vi "pm.vi"() -> ()   [LabVIEW 2017]
uses:
  lowest_col.vi
  index.vi
panel:
  out "String":string
  out "Numeric 2":dbl
  out "Numeric":dbl
  in  "Array":dbl[][](array[numeric])
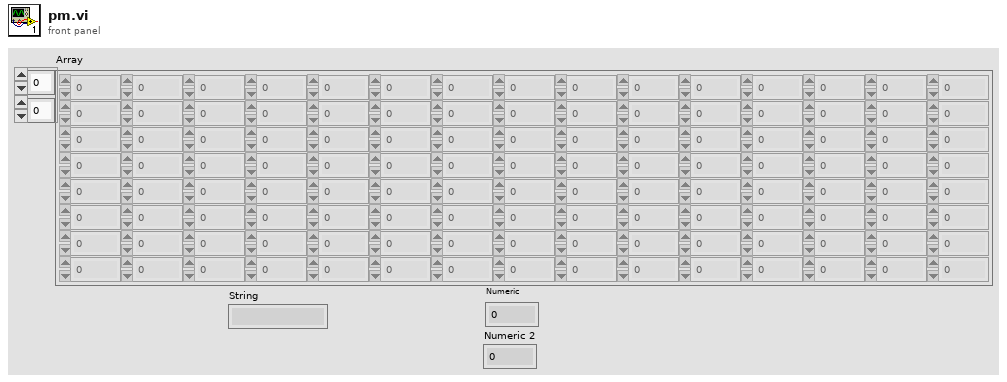
[diagram p1: front panel]
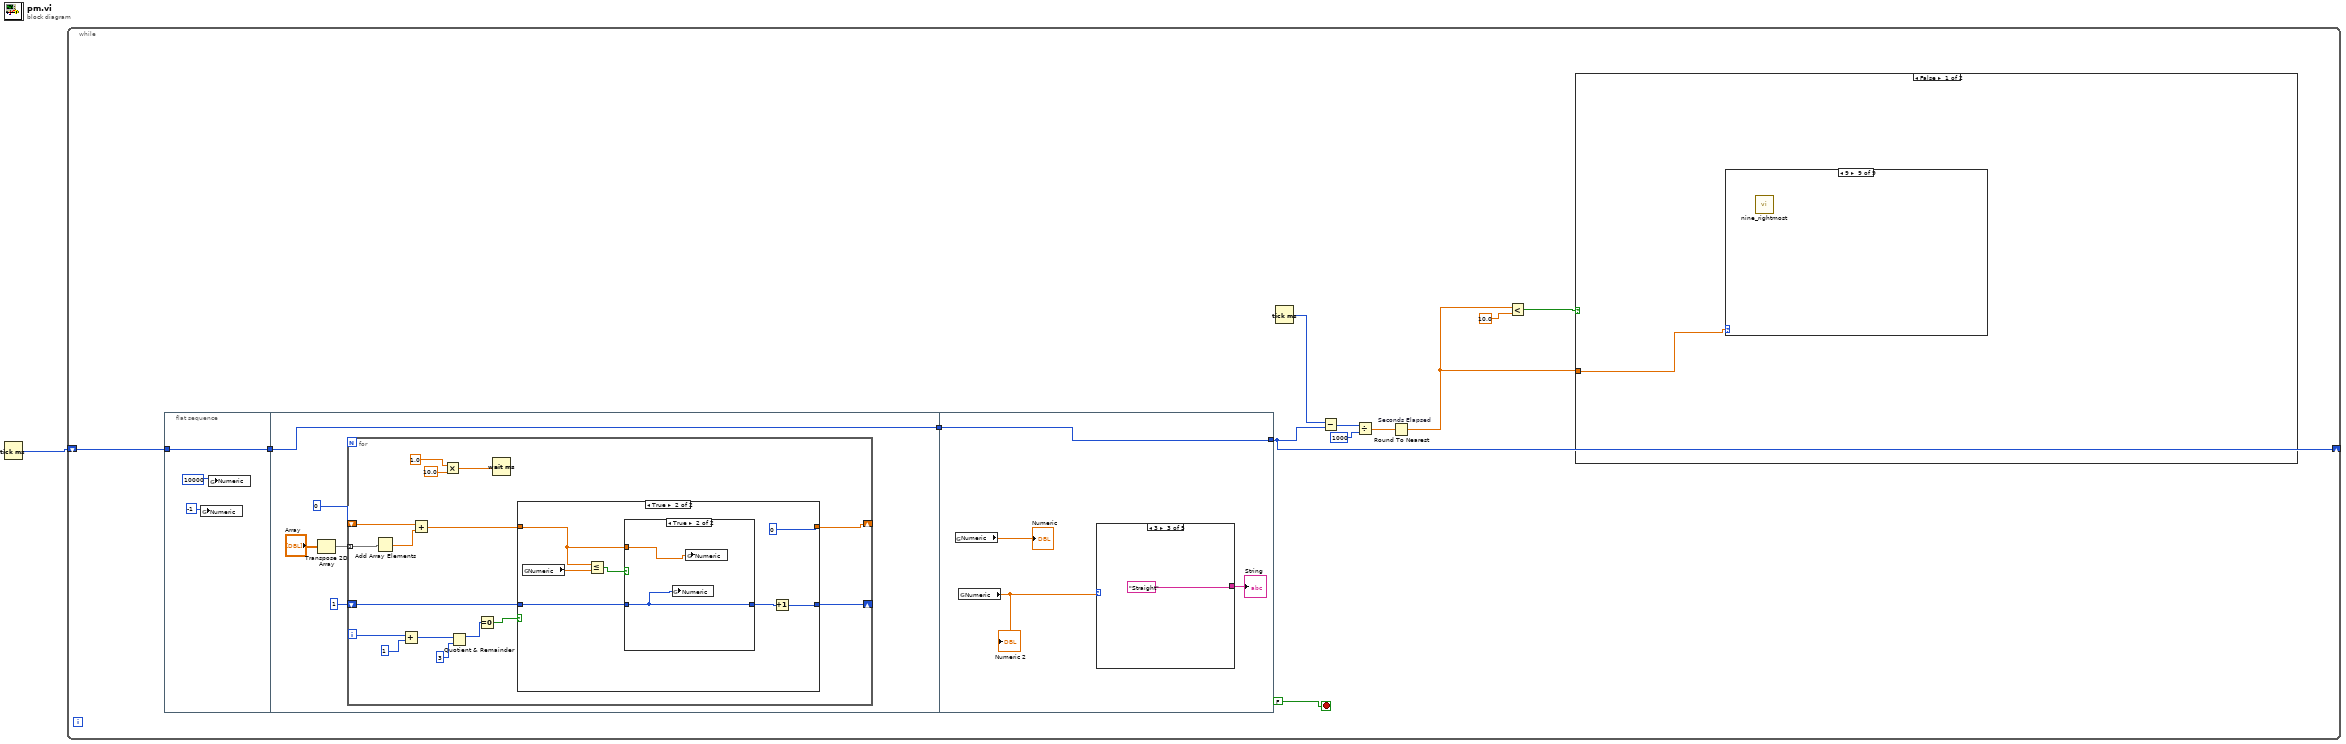
[diagram p0: block diagram]
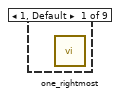
[diagram p2: hidden frame]
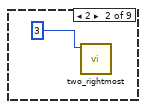
[diagram p3: hidden frame]
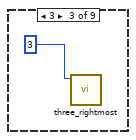
[diagram p4: hidden frame]
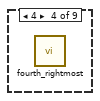
[diagram p5: hidden frame]
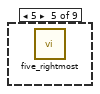
[diagram p6: hidden frame]
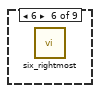
[diagram p7: hidden frame]
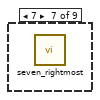
[diagram p8: hidden frame]
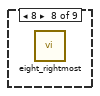
[diagram p9: hidden frame]
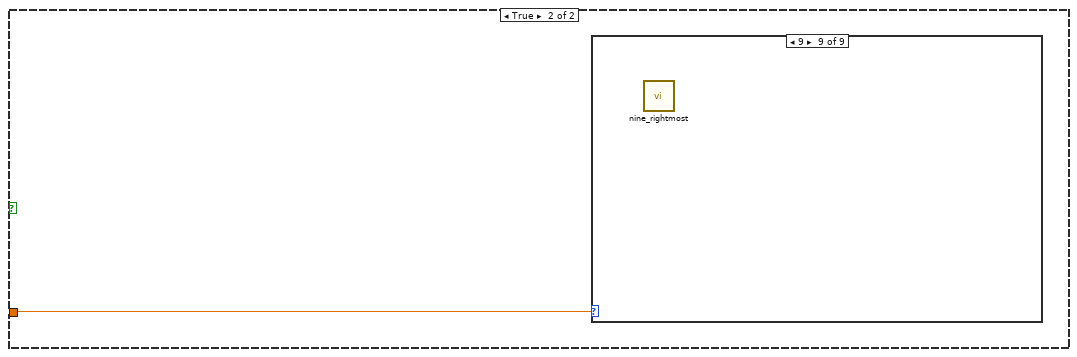
[diagram p10: hidden frame]
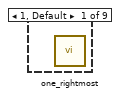
[diagram p11: hidden frame]
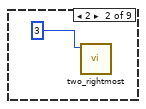
[diagram p12: hidden frame]
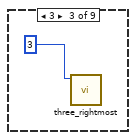
[diagram p13: hidden frame]
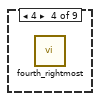
[diagram p14: hidden frame]
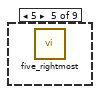
[diagram p15: hidden frame]
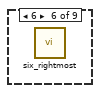
[diagram p16: hidden frame]
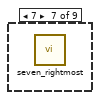
[diagram p17: hidden frame]
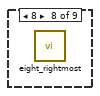
[diagram p18: hidden frame]
diagram:
  n1 = Tick Count (ms)() -> (millisecond timer value=w1:u32)
  n2 = while {
    shift-right: [w8] -> _
    shift-left: w1 -> [w10]
    stop <- FALSE stop-if-true
    n3 = flat-sequence {
      tunnel: [w20] -> w11
      tunnel: w10 -> [w20]
      tunnel: [w23] -> w12
      tunnel: w11 -> [w23]
      tunnel: [w56] -> w8
      tunnel: w12 -> [w56]
      frame #0 {
        n4 = global write "index.vi" "Numeric"(-1) -> ()
        n5 = global write "lowest_col.vi" "Numeric"(10000) -> ()
      }
      frame #1 {
        n6 = Transpose 2D Array(2D array="Array") -> (transposed array=w26:dbl[][])
        n7 = for {
          tunnel: w26 -> [w41] mode=indexing
          shift-right: [w31] -> _
          shift-left: 0 -> [w39]
          shift-right: [w28] -> _
          shift-left: 1 -> [w29]
          i -> [w38]
          n8 = Add Array Elements(numeric array=w41) -> (sum=w40:dbl)
          n9 = Add(x=w38, y=1) -> (x+y=w36:i32)
          n10 = Add(x=w39, y=w40) -> (x+y=w32:dbl)
          n11 = Multiply(x=1.0 ("number (0 to 1)"), y=10.0) -> (x*y=w42:dbl)
          n12 = Quotient & Remainder(x=w36, y=3) -> (x-y*floor(x/y)=w34:i32)  [unwired: 1 out]
          n13 = Equal To 0?(x=w34) -> (x = 0?=w33:bool)
          n14 = Wait (ms)(milliseconds to wait=w42) -> ()  [unwired: 1 out]
          n15 = case shown="True" w33 {
            tunnel: w32 -> [w45 w49]
            tunnel: [w45 0] -> w31
            tunnel: w29 -> [w44 w48]
            tunnel: [w44 w46] -> w28
            frame False {
            }
            frame True {
              n16 = global read "lowest_col.vi" "Numeric"() -> (w51:dbl)
              n17 = Less Or Equal?(x=w49, y=w51) -> (x <= y?=w50:bool)
              n18 = case shown="True" w50 {
                tunnel: w49 -> [_ w55]
                tunnel: w48 -> [w53 w54]
                tunnel: [w53 w54] -> w47
                frame False {
                }
                frame True {
                  n19 = global write "index.vi" "Numeric"(w54) -> ()
                  n20 = global write "lowest_col.vi" "Numeric"(w55) -> ()
                }
              }
              n21 = Increment(x=w47) -> (x+1=w46:i32)
            }
          }
        }
      }
      frame #2 {
        n22 = global read "lowest_col.vi" "Numeric"() -> (→"Numeric":dbl)
        n23 = global read "index.vi" "Numeric"() -> (w58:dbl)
        "Numeric 2" <- w58
        n24 = case shown="3" w58 {
          tunnel: ["Hard Left" "Soft Left" "Straight" "Soft Right" "Hard Right"] -> w57
          frame 1, Default {
          }
          frame 2 {
          }
          frame 3 {
          }
          frame 4 {
          }
          frame 5 {
          }
        }
        "String" <- w57
      }
    }
    n25 = Tick Count (ms)() -> (millisecond timer value=w9:u32)
    n26 = Subtract(x=w9, y=w8) -> (x-y=w7:u32)
    n27 = Divide(x=w7, y=u32 1000) -> (x/y=w5:dbl)
    n28 = Round To Nearest "Seconds Elapsed"(number=w5) -> (nearest integer value=w2:dbl)
    n29 = Less?(x=w2, y=10.0 ("nearest integer value")) -> (x < y?=w3:bool)
    n30 = case shown="False" w3 {
      tunnel: w2 -> [w14 w17]
      frame False {
        n31 = case shown="9" w14 {
          frame 1, Default {
            n32 = call "one_rightmost.vi"() -> ()  [unwired: 12 in]
          }
          frame 2 {
            n33 = call "two_rightmost.vi"("Numeric"=3) -> ()  [unwired: 11 in]
          }
          frame 3 {
            n34 = call "three_rightmost.vi"("Numeric"=3) -> ()  [unwired: 11 in]
          }
          frame 4 {
            n35 = call "fourth_rightmost.vi"() -> ()  [unwired: 12 in]
          }
          frame 5 {
            n36 = call "five_rightmost.vi"() -> ()  [unwired: 12 in]
          }
          frame 6 {
            n37 = call "six_rightmost.vi"() -> ()  [unwired: 12 in]
          }
          frame 7 {
            n38 = call "seven_rightmost.vi"() -> ()  [unwired: 12 in]
          }
          frame 8 {
            n39 = call "eight_rightmost.vi"() -> ()  [unwired: 12 in]
          }
          frame 9 {
            n40 = call "nine_rightmost.vi"() -> ()  [unwired: 12 in]
          }
        }
      }
      frame True {
        n41 = case shown="9" w17 {
          frame 1, Default {
            n42 = call "one_rightmost.vi"() -> ()  [unwired: 12 in]
          }
          frame 2 {
            n43 = call "two_rightmost.vi"("Numeric"=3) -> ()  [unwired: 11 in]
          }
          frame 3 {
            n44 = call "three_rightmost.vi"("Numeric"=3) -> ()  [unwired: 11 in]
          }
          frame 4 {
            n45 = call "fourth_rightmost.vi"() -> ()  [unwired: 12 in]
          }
          frame 5 {
            n46 = call "five_rightmost.vi"() -> ()  [unwired: 12 in]
          }
          frame 6 {
            n47 = call "six_rightmost.vi"() -> ()  [unwired: 12 in]
          }
          frame 7 {
            n48 = call "seven_rightmost.vi"() -> ()  [unwired: 12 in]
          }
          frame 8 {
            n49 = call "eight_rightmost.vi"() -> ()  [unwired: 12 in]
          }
          frame 9 {
            n50 = call "nine_rightmost.vi"() -> ()  [unwired: 12 in]
          }
        }
      }
    }
  }
